vi "Group Name Prompt.vi"(7 "Prompt":string) -> (1 "Cancelled":bool, 2 "Name":string)   [LabVIEW 2020, in "VolatusGUI.lvlib" / "Historian Charting Manager.lvclass"]
uses:
  Historian Charting Manager.lvclass
  Historian Charting Manager.lvclass/Historian Charting Manager.ctl
panel:
  in  "Cancel":bool
  in  "Accept":bool
  in  "New Name":string
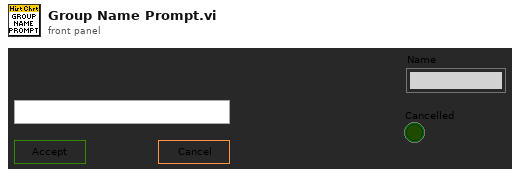
[diagram p1: front panel]
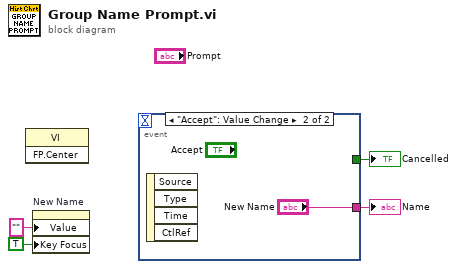
[diagram p0: block diagram]
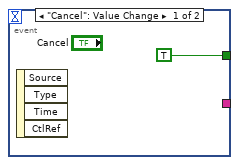
[diagram p2: hidden frame]
diagram:
  n1 = invoke class="VI" method="FP.Center"() -> ()  [unwired: 3 in, 3 out]
  n2 = property on="New Name" class="Str"("Value"="" ("New Name"), "Key Focus"=TRUE) -> ()  [unwired: 2 in, 2 out]
  n3 = event shown="[1] \"Accept\": Value Change" {
    selector: _ -> [_ _]
    dyn-events: _ -> [_ _]
    timeout: _ -> [_ _]
    tunnel: [TRUE _] -> w2
    tunnel: [_ "New Name"] -> w1
    event "Cancel": Value Change {
      n4 = event-data() -> ()  [unwired: 1 in, 4 out]
    }
    event "Accept": Value Change {
      n5 = event-data() -> ()  [unwired: 1 in, 4 out]
    }
  }
  "Cancelled" <- w2
  "Name" <- w1
